vi "Lift.vi"(0 "left encoder":dbl, 1 "right encoder":dbl, 4 "move to distance":dbl, 8 "left output range":cluster{"output high":dbl, "output low":dbl}={"output high"=100.0, "output low"=-100.0} {"output low" format="%.2f"; "output high" format="%.2f"}, 9 "left PID gains":T1={"proportional gain (Kc)"=1.0, "integral time (Ti, min)"=0.01, "derivative time (Td, min)"=0.0} {"derivative time (Td, min)" format="%.3f"; "integral time (Ti, min)" format="%.3f"; "proportional gain (Kc)" format="%.3f"}, 10 "constant":dbl, 12 "right output range":cluster{"output high":dbl, "output low":dbl}={"output high"=100.0, "output low"=-100.0} {"output low" format="%.2f"; "output high" format="%.2f"}, 13 "right PID gains":T1={"proportional gain (Kc)"=1.0, "integral time (Ti, min)"=0.01, "derivative time (Td, min)"=0.0} {"derivative time (Td, min)" format="%.3f"; "integral time (Ti, min)" format="%.3f"; "proportional gain (Kc)" format="%.3f"}) -> (14 "lift motor left":dbl=-0.25, 16 "lift motor right":dbl=0.5)   [LabVIEW 2014]
uses:
  <vilib>/addons/control/pid/pid.llb/PID (DBL).vi
  <vilib>/addons/control/pid/NI_PID_pid.lvlib
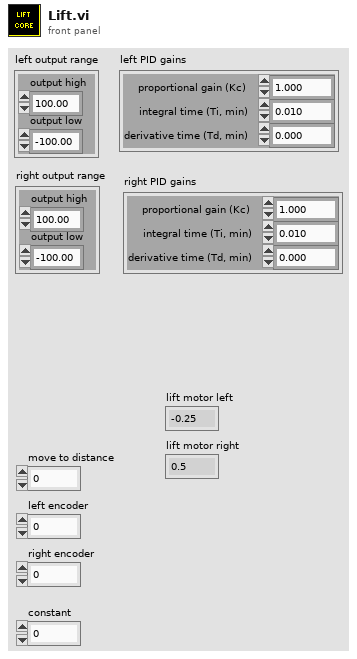
[diagram p1: front panel]
types:
  T1 = cluster{"proportional gain (Kc)":dbl, "integral time (Ti, min)":dbl, "derivative time (Td, min)":dbl}
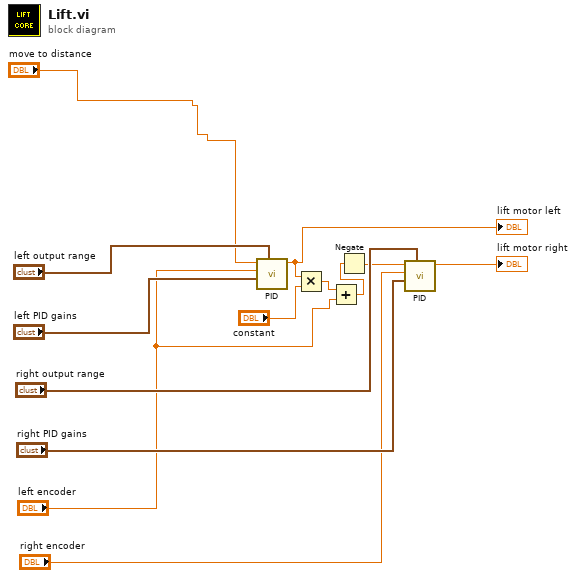
[diagram p0: block diagram]
diagram:
  n1 = call-poly <vilib>:"PID.vi"("output range"="left output range", "PID gains"="left PID gains", "process variable"="left encoder", "setpoint"="move to distance") -> ("output"=w6:dbl)  [unwired: 6 in, 1 out]
  "lift motor left" <- w6
  n2 = Multiply(x=w6, y="constant") -> (x*y=w2:dbl)
  n3 = Add(x=w2, y="left encoder") -> (x+y=w4:dbl)
  n4 = Negate(x=w4) -> (-x=w8:dbl)
  n5 = call-poly <vilib>:"PID.vi"("output range"="right output range", "PID gains"="right PID gains", "process variable"="right encoder", "setpoint"=w8) -> ("output"=→"lift motor right":dbl)  [unwired: 6 in, 1 out]
